vi "set startup speed.vi"(8 "error in (no error)":errorcluster, 11 "focus in":refnum<class "focus.lvclass">) -> (0 "error out":errorcluster, 3 "focus out":refnum<class "focus.lvclass">)   [LabVIEW 2012, in "focus.lvclass"]
uses:
  focus.lvclass
  focus.lvclass/focus.ctl
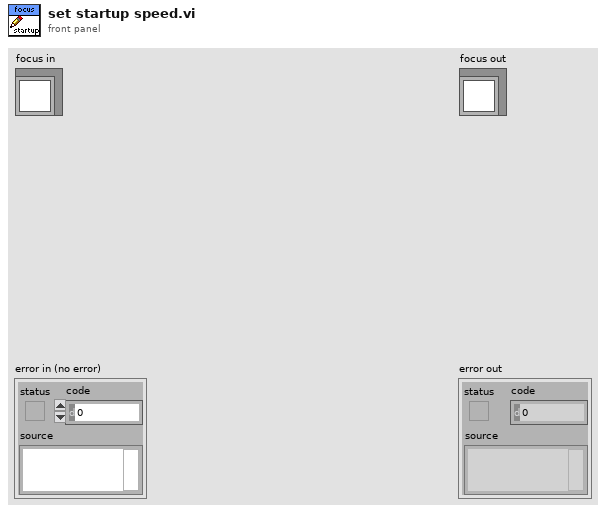
[diagram p1: front panel]
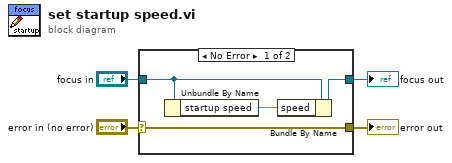
[diagram p0: block diagram]
diagram:
  n1 = case shown="No Error" "error in (no error)" {
    selector: "error in (no error)" -> [w8 w10]
    tunnel: [w8 w10] -> w3
    tunnel: [w6 w9] -> w1
    tunnel: "focus in" -> [w7 w9]
    frame No Error {
      n2 = Unbundle By Name(w7) -> ("startup speed"=w5:dbl[unit])
      n3 = Bundle By Name(cluster=w7, "speed"=w5) -> (w6:refnum<class "focus.lvclass">)
    }
    frame Error {
    }
  }
  "error out" <- w3
  "focus out" <- w1
